vi "ParseVTCommand2.vi"(10 "read buffer":u8[](array[numeric])) -> (0 "location":i32, 1 "Rest":string, 2 "VT data":string, 3 "VT Cmd":string, 5 "remaining":u8[](array[numeric]))   [LabVIEW 2020]
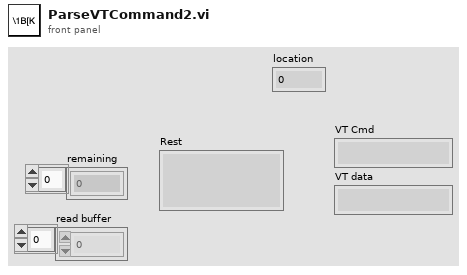
[diagram p1: front panel]
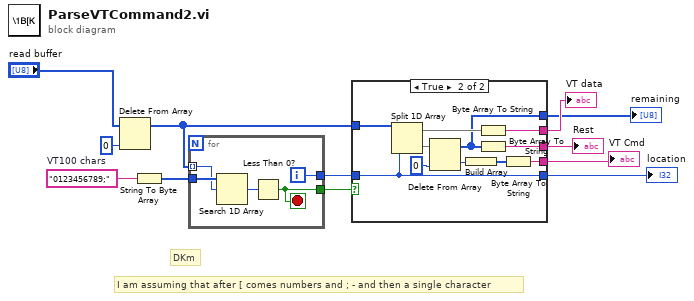
[diagram p0: block diagram]
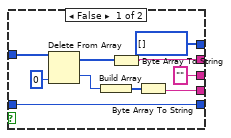
[diagram p2: hidden frame]
diagram:
  w9 = "0123456789;"  # VT100 chars
  # "I am assuming that after [ comes numbers and ; - and then a single character"
  # "DKm"
  n1 = Delete From Array(array="read buffer", index=0) -> (array with subset deleted=w5:u8[])  [unwired: 1 in, 1 out]
  n2 = String To Byte Array(string=w9) -> (unsigned byte array=w10:u8[])
  n3 = for {
    tunnel: w10 -> [w17]
    tunnel: w5 -> [w16] mode=indexing
    tunnel: [w14] -> w6
    tunnel: [w13] -> w8
    i -> [w14]
    stop <- w13 stop-if-true
    n4 = Search 1D Array(1D array=w17, element=w16) -> (index of element=w15:i32)  [unwired: 1 in]
    n5 = Less Than 0?(x=w15) -> (x < 0?=w13:bool)
  }
  n6 = case shown="True" w8 {
    tunnel: [w19 w38] -> w12
    tunnel: ["" ("string") w36] -> w11
    tunnel: w5 -> [w25 w34]
    tunnel: [w26 w33] -> w7
    tunnel: w6 -> [w26 w33]
    tunnel: [w21 w30] -> w3
    tunnel: [u8[] [] w28] -> w1
    frame False {
      n7 = Delete From Array(array=w25, index=0) -> (deleted portion=w22:u8, array with subset deleted=w20:u8[])  [unwired: 1 in]
      n8 = Build Array(w22) -> (w23:u8[])
      n9 = Byte Array To String(unsigned byte array=w20) -> (string=w19:string)
      n10 = Byte Array To String(unsigned byte array=w23) -> (string=w21:string)
    }
    frame True {
      n11 = Split 1D Array(array=w34, index=w33) -> (first subarray=w37:u8[], second subarray=w35:u8[])
      n12 = Delete From Array(array=w35, index=0) -> (deleted portion=w29:u8, array with subset deleted=w28:u8[])  [unwired: 1 in]
      n13 = Build Array(w29) -> (w31:u8[])
      n14 = Byte Array To String(unsigned byte array=w37) -> (string=w38:string)
      n15 = Byte Array To String(unsigned byte array=w28) -> (string=w36:string)
      n16 = Byte Array To String(unsigned byte array=w31) -> (string=w30:string)
    }
  }
  "VT data" <- w12
  "Rest" <- w11
  "location" <- w7
  "VT Cmd" <- w3
  "remaining" <- w1
